vi "Get Resource ID.vi"(11 "GPIO in":refnum<class "GPIO.lvclass">) -> (2 "Resource ID":string)   [LabVIEW 2020, in "CTI.lvlib" / "GPIO.lvclass"]
uses:
  GPIO.lvclass
  GPIO.lvclass/GPIO.ctl
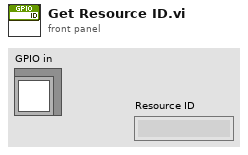
[diagram p1: front panel]
types:
  T1 = typedef "CTI.lvlib/GPIO Number.ctl" = i8
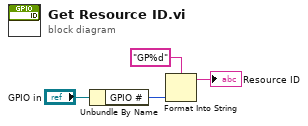
[diagram p0: block diagram]
diagram:
  n1 = Unbundle By Name("GPIO in") -> ("GPIO #"=w3:T1)
  n2 = Format Into String(format string="GP%d", w3) -> (resulting string=→"Resource ID":string)  [unwired: 2 in, 1 out]
